vi "TestInitial.vi"() -> ()   [LabVIEW 2024]
uses:
  <vilib>/numeric/Random Number (Range) U64.vi
  <vilib>/numeric/sub_Random U32.vi
panel:
  out "Boolean 2":bool
  in  "Boolean":bool
  out "number":u64
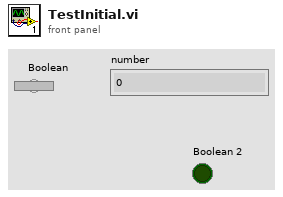
[diagram p1: front panel]
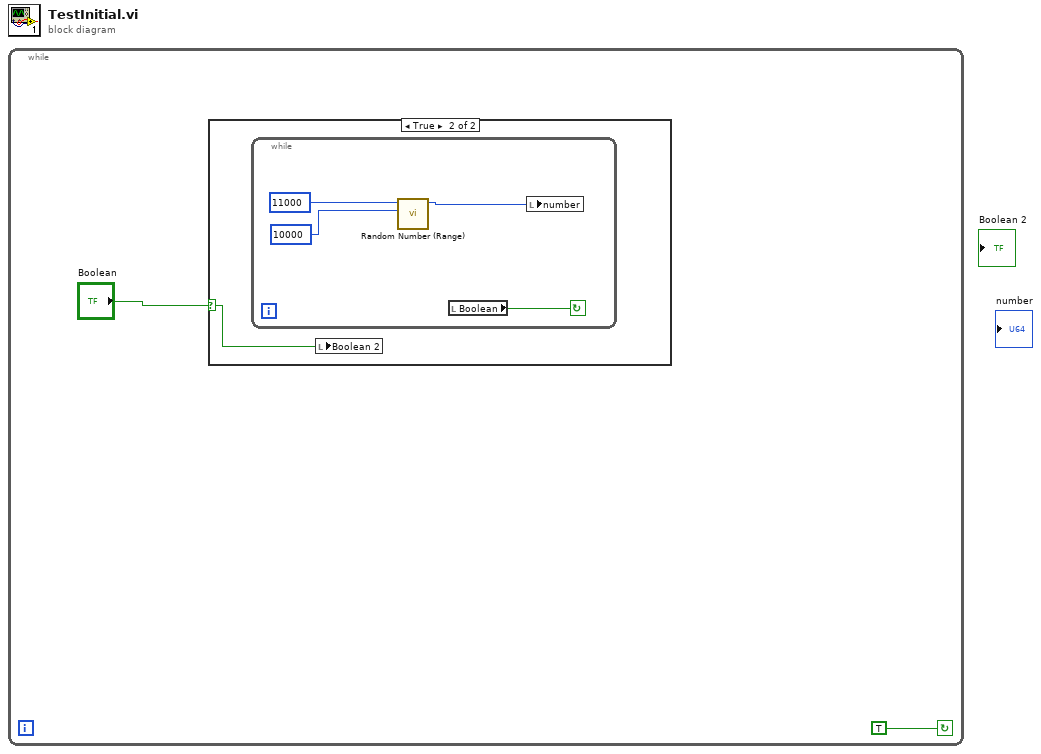
[diagram p0: block diagram]
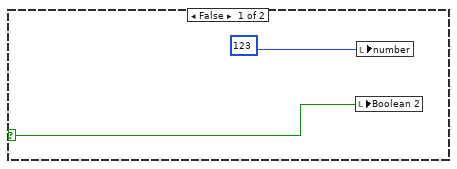
[diagram p2: hidden frame]
diagram:
  n1 = while {
    stop <- TRUE continue-if-true
    n2 = case shown="True" "Boolean" {
      selector: "Boolean" -> [w3 w5]
      frame False {
        n3 = local write "Boolean 2"(w3) -> ()
        n4 = local write "number"(u64 123 ("number")) -> ()
      }
      frame True {
        n5 = while {
          stop <- w7 continue-if-true
          n6 = call-poly <vilib>:"Random Number (Range).vi"("lower bound (0)"=u64 10000, "upper bound (100)"=u64 11000) -> ("number"=w6:u64)  [unwired: 9 in]
          n7 = local read "Boolean"() -> (w7:bool)
          n8 = local write "number"(w6) -> ()
        }
        n9 = local write "Boolean 2"(w5) -> ()
      }
    }
  }
